vi "Generator.vi"(0 "采样点数":i32, 1 "采样频率（Hz）":sgl, 2 "幅度（V）":sgl, 3 "频率（Hz）":dbl, 4 "初始相位":sgl, 5 "直流偏移":sgl, 6 "占空比（%）":i8, 7 "波形选择":enum16{"正弦波", "三角波", "方波", "锯齿波"}(ring), 8 "延时选择":i16) -> (14 "监视器":waveform(dbl)(graph))   [LabVIEW 2022 SP3]
uses:
  <vilib>/Analysis/NI_AALBase.lvlib
panel:
  out "波形数据":waveform(dbl)
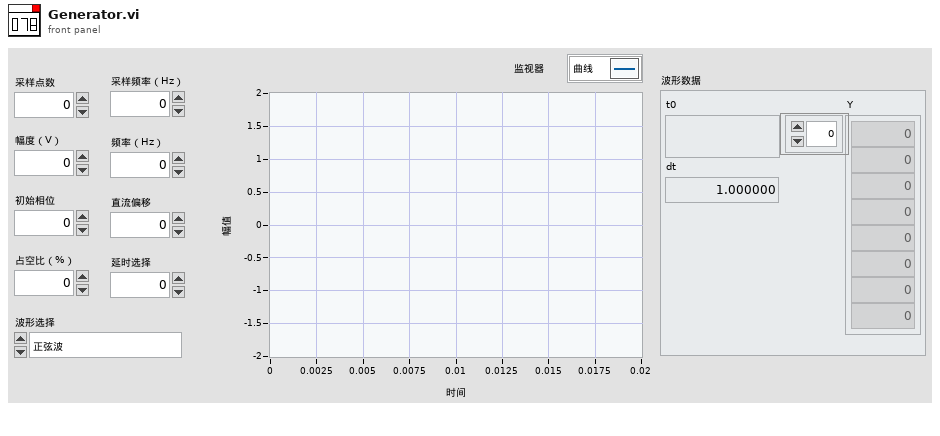
[diagram p1: front panel]
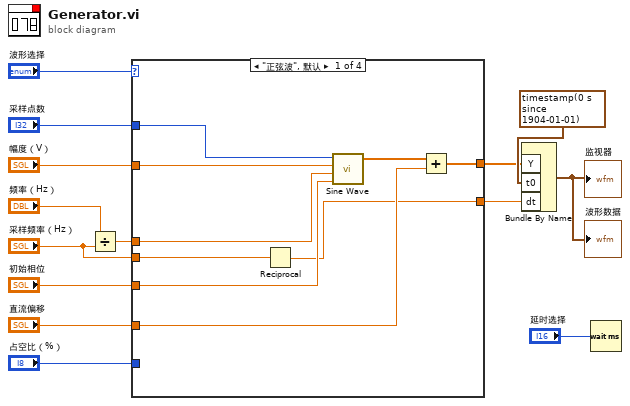
[diagram p0: block diagram]
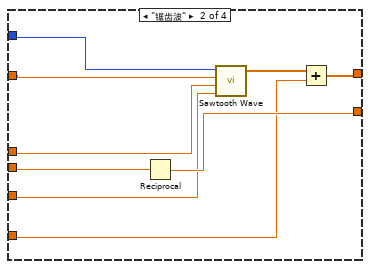
[diagram p2: hidden frame]
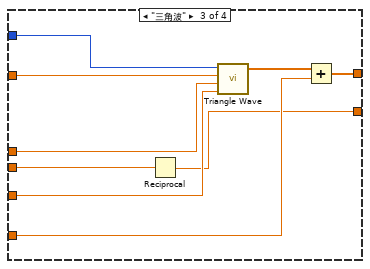
[diagram p3: hidden frame]
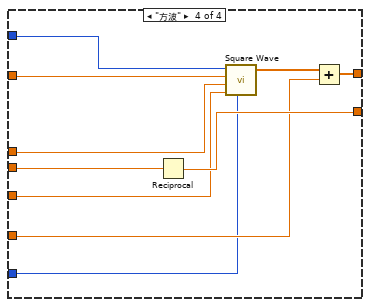
[diagram p4: hidden frame]
diagram:
  n1 = Divide(x="频率（Hz）", y="采样频率（Hz）") -> (x/y=w11:dbl)
  n2 = case shown="\"正弦波\", 默认" "波形选择" {
    tunnel: "初始相位" -> [w23 w28 w36 w47]
    tunnel: "幅度（V）" -> [w22 w24 w39 w43]
    tunnel: "采样点数" -> [w21 w25 w40 w44]
    tunnel: "采样频率（Hz）" -> [w20 w27 w37 w46]
    tunnel: "直流偏移" -> [w19 w29 w35 w48]
    tunnel: [w17 w31 w33 w49] -> w9
    tunnel: [w16 w30 w34 w50] -> w10
    tunnel: w11 -> [w15 w26 w38 w45]
    tunnel: "占空比（%）" -> [_ _ _ w42]
    frame "正弦波", Default {
      n3 = Reciprocal(x=w20) -> (1/x=w16:sgl)
      n4 = call <vilib>:"Sine Wave.vi"("samples"=w21, "amplitude"=w22, "frequency"=w15, "phase in"=w23) -> ("sine wave"=w18:dbl[])  [unwired: 1 in, 2 out]
      n5 = Add(x=w18, y=w19) -> (x+y=w17:dbl[])
    }
    frame "锯齿波" {
      n6 = Reciprocal(x=w27) -> (1/x=w30:sgl)
      n7 = call <vilib>:"Sawtooth Wave.vi"("samples"=w25, "amplitude"=w24, "frequency"=w26, "phase in"=w28) -> ("sawtooth wave"=w32:dbl[])  [unwired: 1 in, 2 out]
      n8 = Add(x=w32, y=w29) -> (x+y=w31:dbl[])
    }
    frame "三角波" {
      n9 = Reciprocal(x=w37) -> (1/x=w34:sgl)
      n10 = call <vilib>:"Triangle Wave.vi"("samples"=w40, "amplitude"=w39, "frequency"=w38, "phase in"=w36) -> ("triangle wave"=w41:dbl[])  [unwired: 1 in, 2 out]
      n11 = Add(x=w41, y=w35) -> (x+y=w33:dbl[])
    }
    frame "方波" {
      n12 = Reciprocal(x=w46) -> (1/x=w50:sgl)
      n13 = call <vilib>:"Square Wave.vi"("samples"=w44, "amplitude"=w43, "frequency"=w45, "duty cycle (%)"=w42, "phase in"=w47) -> ("square wave"=w51:dbl[])  [unwired: 1 in, 2 out]
      n14 = Add(x=w51, y=w48) -> (x+y=w49:dbl[])
    }
  }
  n15 = Bundle By Name("Y"=w9, "t0"=timestamp(0 s since 1904-01-01), "dt"=w10) -> (→"监视器" →"波形数据":waveform(dbl))  [unwired: 1 in]
  n16 = Wait (ms)(milliseconds to wait="延时选择") -> ()  [unwired: 1 out]
